vi "Tosca-Setup Visual Display.vi"() -> (1 "cancelled?":bool)   [LabVIEW 2020]
uses:
  epl-vi-lib/Utility VIs/Buttons/KCheckmarkBoolean 2.ctl
panel:
  in  "Monitor":i32=1 min=1
  in  "close event":refnum<user-event>
  in  "Background":dbl=1.0 min=0.0 max=1.0
  in  "Open now":bool
  in  "Close":bool
  in  "Location":T1(ring)
  in  "Photodiode square":i16=1
  in  "Open at startup":T2
  in  "Init PTB":bool
  in  "Distance (inches)":dbl=1.0
  in  "Tab":enum32{"Page 1"}(tab)
  in  "Fullscreen":T2 caption="Open window at startup"
  in  "rect":T3
  in  "Diagonal size (inches)":dbl=1.0
  in  "Use PsychToolbox":T2
  in  "Port":i32
  in  "IP Address":string
  out "Ping result":bool
  in  "Ping":bool
  in  "Release PTB":bool
  # "Right Primary"
  # "Right Primary"
  # "Right Primary"
  # "Right Primary"
  # "Laser enable"
  # "Right Primary"
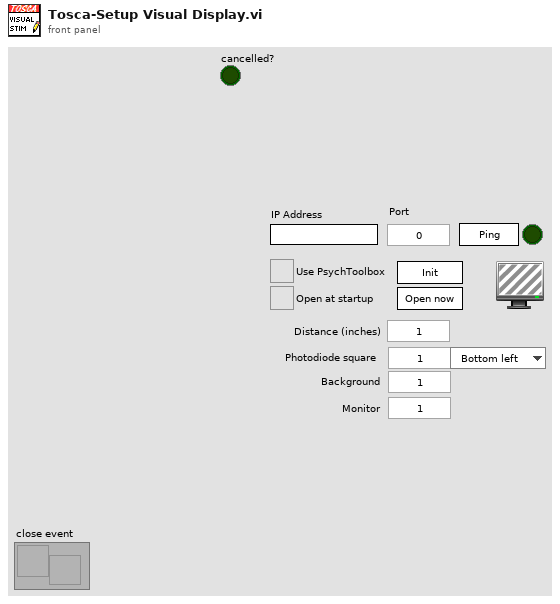
[diagram p1: front panel]
types:
  T1 = enum16{"Bottom left", "Top left", "Top right", "Bottom right"}
  T2 = typedef "KCheckmarkBoolean 2.ctl" = bool
  T3 = cluster{"Left":i32, "Top":i32, "Width":i32, "Height":i32}
  T4 = typedef "Tosca-Visual Display Settings.ctl" = cluster{"Use PTB":bool, "IP Address":string, "Port":i32, "rect":cluster{"left":i16, "top":i16, "width":i16, "height":i16}, "Full screen":bool, "Open at start":bool, "Monitor":i32, "Monitor size (in)":dbl, "Monitor dist (in)":dbl, "Photodiode Square":cluster{"size":i16, "location":enum16{"Bottom Left", "Top Left", "Top Right", "Bottom Right"}}, "Background":dbl}
  T5 = enum16{"Bottom Left", "Top Left", "Top Right", "Bottom Right"}
  T6 = cluster{"left":i16, "top":i16, "width":i16, "height":i16}
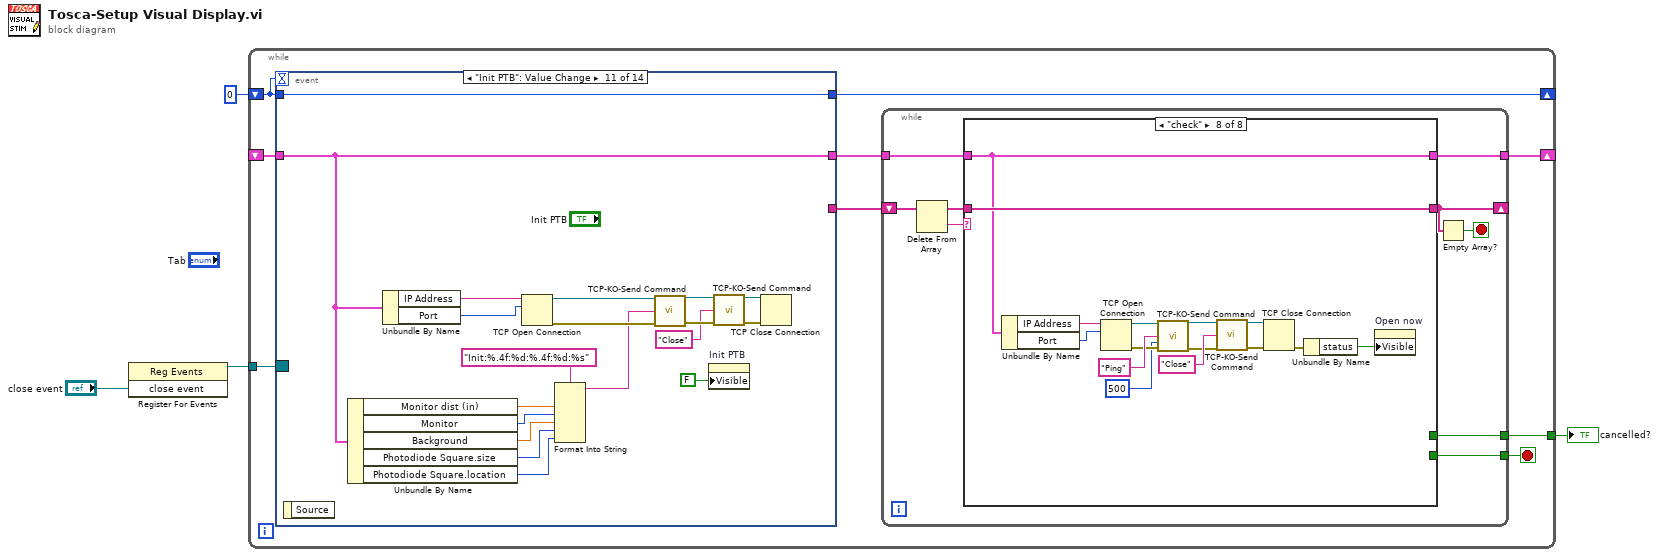
[diagram p0: block diagram]
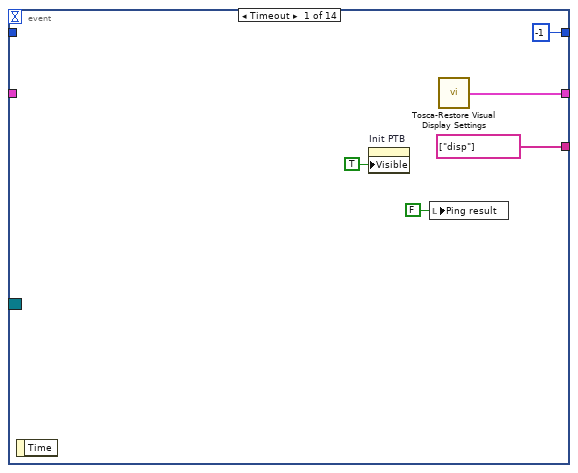
[diagram p2: hidden frame]
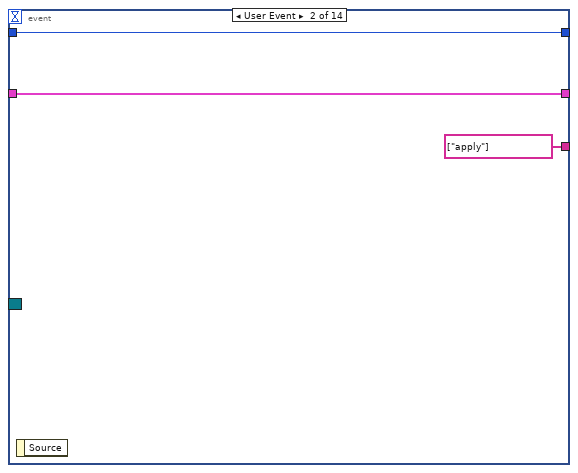
[diagram p3: hidden frame]
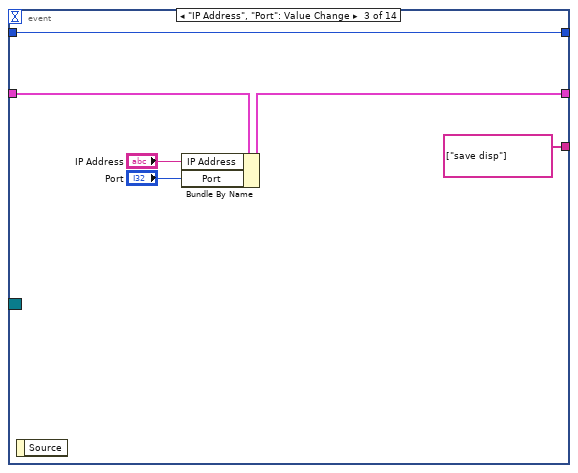
[diagram p4: hidden frame]
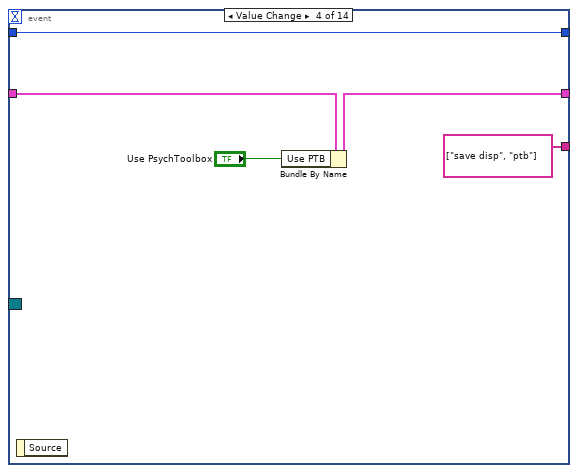
[diagram p5: hidden frame]
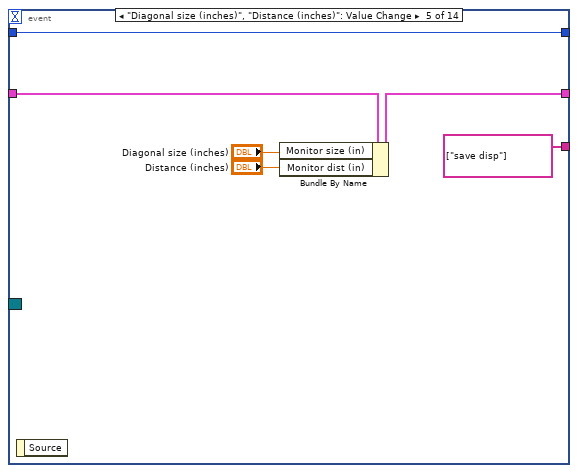
[diagram p6: hidden frame]
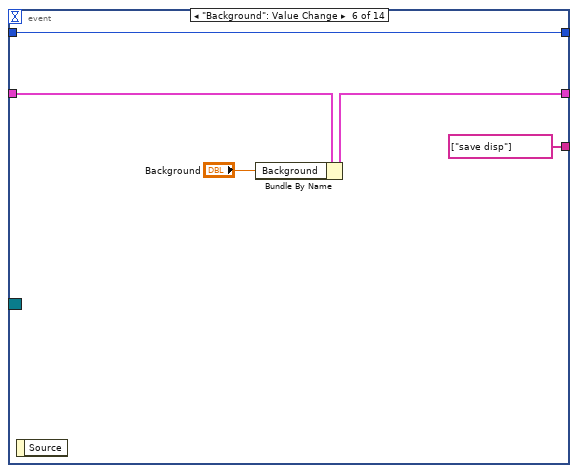
[diagram p7: hidden frame]
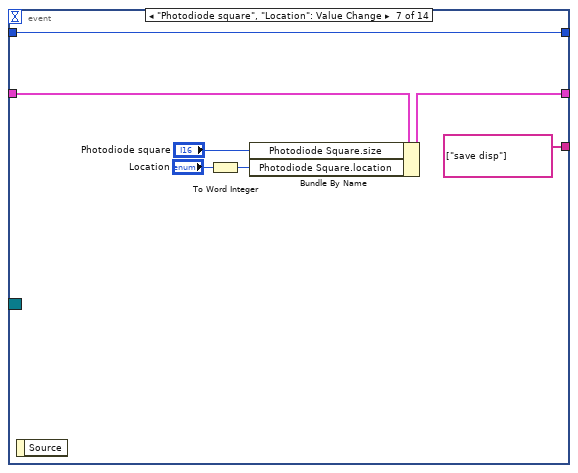
[diagram p8: hidden frame]
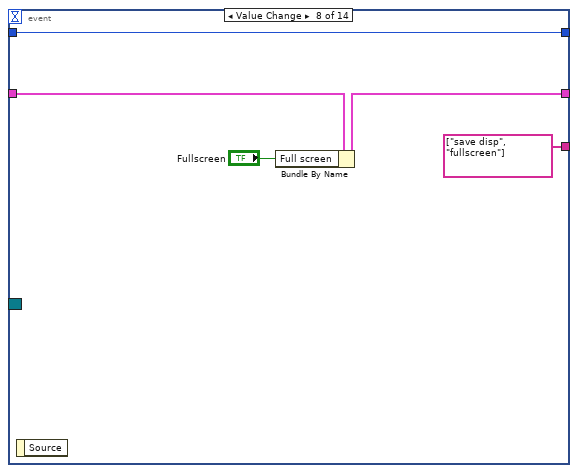
[diagram p9: hidden frame]
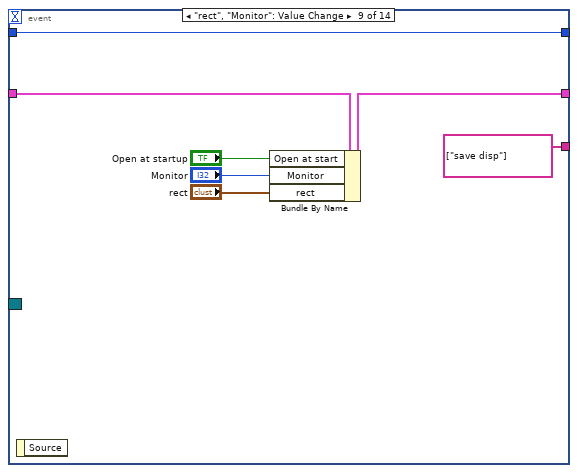
[diagram p10: hidden frame]
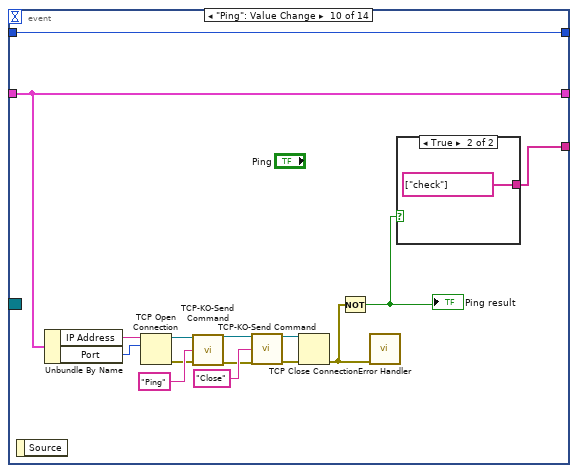
[diagram p11: hidden frame]
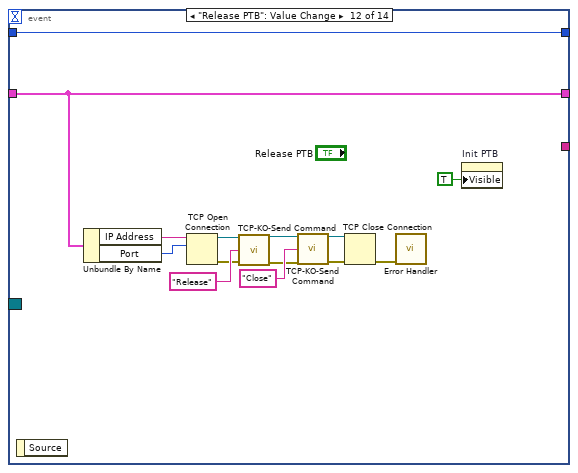
[diagram p13: hidden frame]
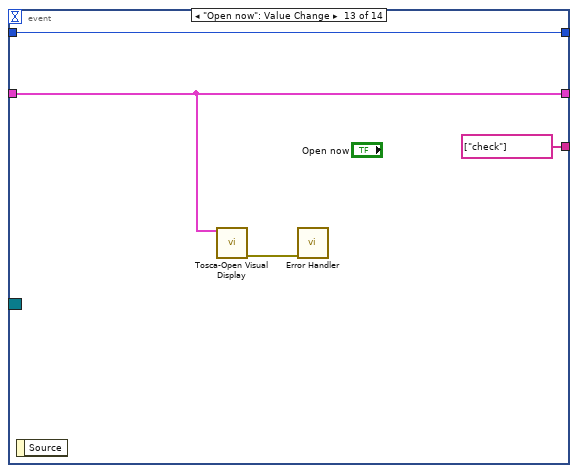
[diagram p14: hidden frame]
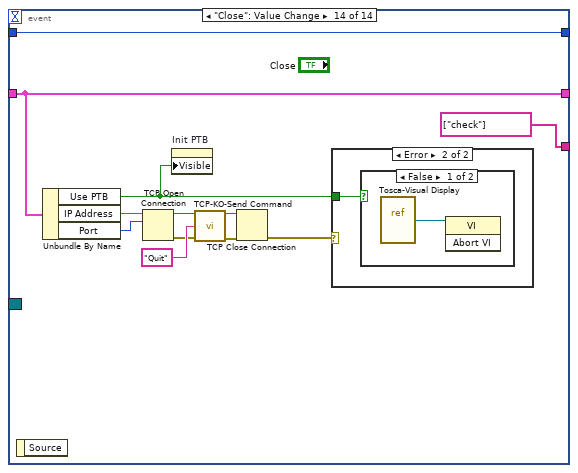
[diagram p15: hidden frame]
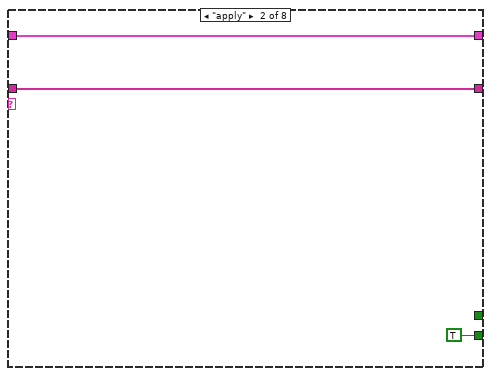
[diagram p19: hidden frame]
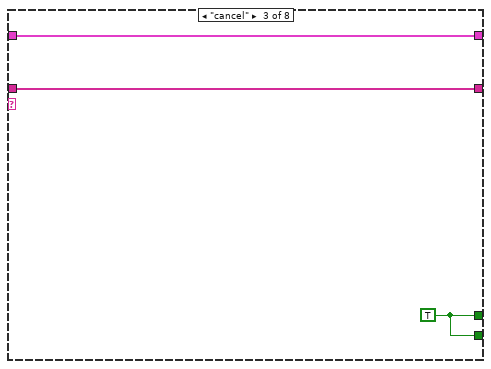
[diagram p20: hidden frame]
diagram:
  n1 = register-events("close event") -> (reference out=w1:refnum<event-registration>)  [unwired: 2 in, 1 out]
  n2 = while {
    shift-right: [w13] -> _
    shift-left: 0 -> [w12]
    tunnel: [w7] -> w3
    shift-right: [w10] -> _
    shift-left: _ -> [w9]
    tunnel: w1 -> [w5]
    stop <- w6 stop-if-true
    n3 = event shown="[10] \"Init PTB\": Value Change" {
      selector: w5 -> [_ _ _ _ _ _ _ _ _ _ _ _ _ _]
      dyn-events: _ -> [_ _ _ _ _ _ _ _ _ _ _ _ _ _]
      timeout: w12 -> [_ _ _ _ _ _ _ _ _ _ _ _ _ _]
      tunnel: [-1 w21 w27 w32 w38 w43 w50 w55 w62 w77 w97 w111 w115 w127] -> w13
      tunnel: w12 -> [_ w21 w27 w32 w38 w43 w50 w55 w62 w77 w97 w111 w115 w127]
      tunnel: [w17 w20 w25 w30 w36 w41 w48 w53 w60 w76 w95 w110 w112 w125] -> w11
      tunnel: w9 -> [_ w20 w26 w31 w37 w42 w49 w54 w61 w76 w95 w110 w112 w125]
      tunnel: [string[] ["disp"] string[] ["apply"] string[] ["save disp"] string[] ["save disp", "ptb"] string[] ["save disp"] string[] ["save disp"] string[] ["save disp"] string[] ["save disp", "fullscreen"] string[] ["save disp"] w74 _ _ string[] ["check"] string[] ["check"]] -> w8
      event Timeout {
        n4 = event-data() -> ()  [unwired: 1 in, 1 out]
        n5 = property on="Init PTB" class="Bool"("Visible"=TRUE) -> ()  [unwired: 2 in, 2 out]
        n6 = local write "Ping result"(FALSE ("Ping result")) -> ()
        n7 = call "Tosca-Restore Visual Display Settings.vi"() -> ("Visual Display Settings"=w17:T4)  [unwired: 14 in, 1 out]
      }
      event User Event {
        n8 = event-data() -> ()  [unwired: 1 in, 1 out]
      }
      event "IP Address", "Port": Value Change {
        n9 = event-data() -> ()  [unwired: 1 in, 1 out]
        n10 = Bundle By Name(cluster=w26, "IP Address"="IP Address", "Port"="Port") -> (w25:T4)
      }
      event Value Change {
        n11 = event-data() -> ()  [unwired: 1 in, 1 out]
        n12 = Bundle By Name(cluster=w31, "Use PTB"="Use PsychToolbox") -> (w30:T4)
      }
      event "Diagonal size (inches)", "Distance (inches)": Value Change {
        n13 = event-data() -> ()  [unwired: 1 in, 1 out]
        n14 = Bundle By Name(cluster=w37, "Monitor size (in)"="Diagonal size (inches)", "Monitor dist (in)"="Distance (inches)") -> (w36:T4)
      }
      event "Background": Value Change {
        n15 = event-data() -> ()  [unwired: 1 in, 1 out]
        n16 = Bundle By Name(cluster=w42, "Background"="Background") -> (w41:T4)
      }
      event "Photodiode square", "Location": Value Change {
        n17 = event-data() -> ()  [unwired: 1 in, 1 out]
        n18 = To Word Integer(number="Location") -> (16bit integer=w44:i16)
        n19 = Bundle By Name(cluster=w49, "Photodiode Square.size"="Photodiode square", "Photodiode Square.location"=w44) -> (w48:T4)
      }
      event Value Change {
        n20 = event-data() -> ()  [unwired: 1 in, 1 out]
        n21 = Bundle By Name(cluster=w54, "Full screen"="Fullscreen") -> (w53:T4)
      }
      event "rect", "Monitor": Value Change {
        n22 = event-data() -> ()  [unwired: 1 in, 1 out]
        n23 = Bundle By Name(cluster=w61, "Open at start"="Open at startup", "Monitor"="Monitor", "rect"="rect") -> (w60:T4)
      }
      event "Ping": Value Change {
        n24 = event-data() -> ()  [unwired: 1 in, 1 out]
        n25 = Unbundle By Name(w76) -> ("IP Address"=w69:string, "Port"=w68:i32)
        n26 = TCP Open Connection(address=w69, remote port or service name=w68) -> (connection ID=w73:refnum<k5>, error out=w66:errorcluster)  [unwired: 3 in]
        n27 = call "TCP-KO-Send Command.vi"("connection ID"=w73, "Command"="Ping", "error in (no error)"=w66) -> ("connection ID out"=w72:refnum<k5>, "error out"=w65:errorcluster)  [unwired: 11 in]
        n28 = call "TCP-KO-Send Command.vi"("connection ID"=w72, "Command"="Close", "error in (no error)"=w65) -> ("connection ID out"=w70:refnum<k5>, "error out"=w64:errorcluster)  [unwired: 11 in]
        n29 = TCP Close Connection(connection ID=w70, error in (no error)=w64) -> (error out=w63:errorcluster)  [unwired: 1 in, 1 out]
        n30 = Not(x=w63) -> (.not. x?=w75:bool)
        "Ping result" <- w75
        n31 = call "Error Handler.vi"("error in (no error)"=w63) -> ()  [unwired: 13 in, 2 out]
        n32 = case shown="True" w75 {
          tunnel: [_ string[] ["check"]] -> w74
          frame False {
          }
          frame True {
          }
        }
      }
      event "Init PTB": Value Change {
        n33 = event-data() -> ()  [unwired: 1 in, 1 out]
        n34 = Unbundle By Name(w95) -> ("Monitor dist (in)"=w94:dbl, "Monitor"=w89:i32, "Background"=w92:dbl, "Photodiode Square.size"=w91:i16, "Photodiode Square.location"=w90:T5)
        n35 = Unbundle By Name(w95) -> ("IP Address"=w88:string, "Port"=w87:i32)
        n36 = TCP Open Connection(address=w88, remote port or service name=w87) -> (connection ID=w86:refnum<k5>, error out=w85:errorcluster)  [unwired: 3 in]
        n37 = Format Into String(format string="Init:%.4f:%d:%.4f:%d:%s" ("Command"), w94, w89, w92, w91, w90) -> (resulting string=w84:string)  [unwired: 2 in, 1 out]
        n38 = call "TCP-KO-Send Command.vi"("connection ID"=w86, "Command"=w84, "error in (no error)"=w85) -> ("connection ID out"=w82:refnum<k5>, "error out"=w83:errorcluster)  [unwired: 11 in]
        n39 = property on="Init PTB" class="Bool"("Visible"=FALSE) -> ()  [unwired: 2 in, 2 out]
        n40 = call "TCP-KO-Send Command.vi"("connection ID"=w82, "Command"="Close", "error in (no error)"=w83) -> ("connection ID out"=w79:refnum<k5>, "error out"=w80:errorcluster)  [unwired: 11 in]
        n41 = TCP Close Connection(connection ID=w79, error in (no error)=w80) -> ()  [unwired: 1 in, 2 out]
      }
      event "Release PTB": Value Change {
        n42 = event-data() -> ()  [unwired: 1 in, 1 out]
        n43 = Unbundle By Name(w110) -> ("IP Address"=w100:string, "Port"=w99:i32)
        n44 = TCP Open Connection(address=w100, remote port or service name=w99) -> (connection ID=w108:refnum<k5>, error out=w103:errorcluster)  [unwired: 3 in]
        n45 = call "TCP-KO-Send Command.vi"("connection ID"=w108, "Command"="Release", "error in (no error)"=w103) -> ("connection ID out"=w107:refnum<k5>, "error out"=w102:errorcluster)  [unwired: 11 in]
        n46 = call "TCP-KO-Send Command.vi"("connection ID"=w107, "Command"="Close", "error in (no error)"=w102) -> ("connection ID out"=w105:refnum<k5>, "error out"=w101:errorcluster)  [unwired: 11 in]
        n47 = TCP Close Connection(connection ID=w105, error in (no error)=w101) -> (error out=w98:errorcluster)  [unwired: 1 in, 1 out]
        n48 = call "Error Handler.vi"("error in (no error)"=w98) -> ()  [unwired: 13 in, 2 out]
        n49 = property on="Init PTB" class="Bool"("Visible"=TRUE) -> ()  [unwired: 2 in, 2 out]
      }
      event "Open now": Value Change {
        n50 = event-data() -> ()  [unwired: 1 in, 1 out]
        n51 = call "Tosca-Open Visual Display.vi"("Visual Display Settings"=w112) -> ("error out"=w113:errorcluster)  [unwired: 14 in]
        n52 = call "Error Handler.vi"("error in (no error)"=w113) -> ()  [unwired: 13 in, 2 out]
      }
      event "Close": Value Change {
        n53 = event-data() -> ()  [unwired: 1 in, 1 out]
        n54 = Unbundle By Name(w125) -> ("Use PTB"=w124:bool, "IP Address"=w118:string, "Port"=w117:i32)
        n55 = TCP Open Connection(address=w118, remote port or service name=w117) -> (connection ID=w123:refnum<k5>, error out=w120:errorcluster)  [unwired: 3 in]
        n56 = property on="Init PTB" class="Bool"("Visible"=w124) -> ()  [unwired: 2 in, 2 out]
        n57 = call "TCP-KO-Send Command.vi"("connection ID"=w123, "Command"="Quit", "error in (no error)"=w120) -> ("connection ID out"=w122:refnum<k5>, "error out"=w119:errorcluster)  [unwired: 11 in]
        n58 = TCP Close Connection(connection ID=w122, error in (no error)=w119) -> (error out=w116:errorcluster)  [unwired: 1 in, 1 out]
        n59 = case shown="Error" w116 {
          tunnel: w124 -> [_ w128]
          frame No Error {
          }
          frame Error {
            n60 = case shown="False" w128 {
              frame False {
                n61 = vi-ref "Tosca-Visual Display.vi"() -> (w129:refnum<vi>)
                n62 = invoke class="VI" method="Abort VI"(reference=w129) -> ()  [unwired: 2 in, 3 out]
              }
              frame True {
              }
            }
          }
        }
      }
    }
    n63 = while {
      shift-right: [w135] -> _
      shift-left: w8 -> [w138]
      tunnel: w11 -> [w133]
      tunnel: [w132] -> w10
      tunnel: [w131] -> w7
      tunnel: [w130] -> w6
      stop <- w134 stop-if-true
      n64 = Delete From Array(array=w138) -> (deleted portion=w136:string, array with subset deleted=w137:string[])  [unwired: 2 in]
      n65 = case shown="\"check\"" w136 {
        tunnel: w137 -> [w140 w143 w146 w164 w169 w175 w179 w194]
        tunnel: [w140 w143 w146 w155 w169 w173 w179 w194] -> w135
        tunnel: w133 -> [w139 w142 w145 w163 w166 w174 w178 w192]
        tunnel: [w139 w142 w145 w163 w166 w174 w178 w192] -> w132
        tunnel: [_ _ w144 _ _ _ _ _] -> w131
        tunnel: [_ TRUE w144 _ _ _ _ _] -> w130
        frame "", Default {
        }
        frame "apply" {
        }
        frame "cancel" {
          w144 = TRUE
        }
        frame "disp" {
          n66 = Unbundle By Name(w163) -> ("IP Address"=w162:string, "Port"=w161:i32, "Use PTB"=w160:bool, "Full screen"=w159:bool, "Open at start"=w158:bool, "Monitor"=w157:i32, "rect"=w156:T6, "Monitor size (in)"=w152:dbl, "Monitor dist (in)"=w151:dbl, "Photodiode Square.size"=w150:i16, "Photodiode Square.location"=w149:T5, "Background"=w147:dbl)
          n67 = To Word Integer(number=w149) -> (16bit integer=w148:i16)
          n68 = local write "IP Address"(w162) -> ()
          n69 = local write "Port"(w161) -> ()
          n70 = local write "Use PsychToolbox"(w160) -> ()
          n71 = local write "Fullscreen"(w159) -> ()
          n72 = local write "Open at startup"(w158) -> ()
          n73 = local write "Monitor"(w157) -> ()
          n74 = local write "rect"(w156) -> ()
          n75 = local write "Diagonal size (inches)"(w152) -> ()
          n76 = local write "Distance (inches)"(w151) -> ()
          n77 = local write "Photodiode square"(w150) -> ()
          n78 = local write "Location"(w148) -> ()
          n79 = local write "Background"(w147) -> ()
          n80 = Build Array (concatenate)(w164, "ptb", "fullscreen") -> (w155:string[])
        }
        frame "save disp" {
          n81 = call "Config File Path.vi"("AppName"="Tosca") -> ("Default config file name"=w167:path)
          n82 = call "Write Anything.vi"("Section Name (Name of \"Anything\")"="Visual Display Settings" ("Section Name (Name of \"Anything\")"), "Anything"=w166, "Path (dialog)"=w167) -> ()  [unwired: 7 in, 2 out]
        }
        frame "ptb" {
          n83 = Unbundle By Name(w174) -> ("Use PTB"=w171:bool)
          n84 = Not(x=w171) -> (.not. x?=w172:bool)
          n85 = property on="Tab" class="TabCtl (strict)"("Visible"=w172) -> ()  [unwired: 2 in, 2 out]
          n86 = property on="Release PTB" class="Bool"("Visible"=w171) -> ()  [unwired: 2 in, 2 out]
          n87 = property on="Init PTB" class="Bool"("Visible"=w171) -> ()  [unwired: 2 in, 2 out]
          n88 = Build Array (concatenate)(w175, "check" ("String")) -> (w173:string[])
        }
        frame "fullscreen" {
          n89 = Unbundle By Name(w178) -> ("Full screen"=w177:bool)
          n90 = Not(x=w177) -> (.not. x?=w176:bool)
          n91 = property on="rect" class="Clust (strict)"("Visible"=w176) -> ()  [unwired: 2 in, 2 out]
        }
        frame "check" {
          n92 = Unbundle By Name(w192) -> ("IP Address"=w182:string, "Port"=w181:i32)
          n93 = TCP Open Connection(address=w182, remote port or service name=w181) -> (connection ID=w191:refnum<k5>, error out=w186:errorcluster)  [unwired: 3 in]
          n94 = call "TCP-KO-Send Command.vi"("connection ID"=w191, "Command"="Ping", "timeout (ms)"=500, "error in (no error)"=w186) -> ("connection ID out"=w190:refnum<k5>, "error out"=w185:errorcluster)  [unwired: 10 in]
          n95 = call "TCP-KO-Send Command.vi"("connection ID"=w190, "Command"="Close", "error in (no error)"=w185) -> ("connection ID out"=w188:refnum<k5>, "error out"=w184:errorcluster)  [unwired: 11 in]
          n96 = TCP Close Connection(connection ID=w188, error in (no error)=w184) -> (error out=w180:errorcluster)  [unwired: 1 in, 1 out]
          n97 = Unbundle By Name(w180) -> ("status"=w193:bool)
          n98 = property on="Open now" class="Bool"("Visible"=w193) -> ()  [unwired: 2 in, 2 out]
        }
      }
      n99 = Empty Array?(array=w135) -> (empty?=w134:bool)
    }
  }
  "cancelled?" <- w3
